vi "Angle PID.vi"(6 "reinitialize? (F)":bool, 7 "output range":cluster{"output high":dbl, "output low":dbl}={"output high"=100.0, "output low"=-100.0} {"output low" format="%.2f"; "output high" format="%.2f"}, 8 "dt (s)":dbl=-1.0 format="%.3f", 9 "PID gains":T1={"proportional gain (Kc)"=1.0, "integral time (Ti, min)"=0.01, "derivative time (Td, min)"=0.0} {"derivative time (Td, min)" format="%.3f"; "integral time (Ti, min)" format="%.3f"; "proportional gain (Kc)" format="%.3f"}, 10 "process variable":dbl format="%.2f", 11 "setpoint":dbl format="%.2f") -> (0 "dt out (s)":dbl format="%.3f", 3 "output":dbl format="%.2f")   [LabVIEW 2017]
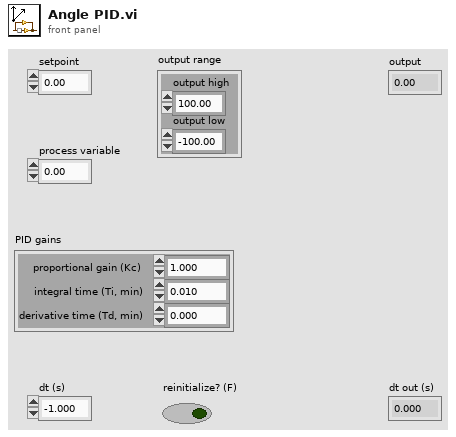
[diagram p1: front panel]
types:
  T1 = cluster{"proportional gain (Kc)":dbl, "integral time (Ti, min)":dbl, "derivative time (Td, min)":dbl}
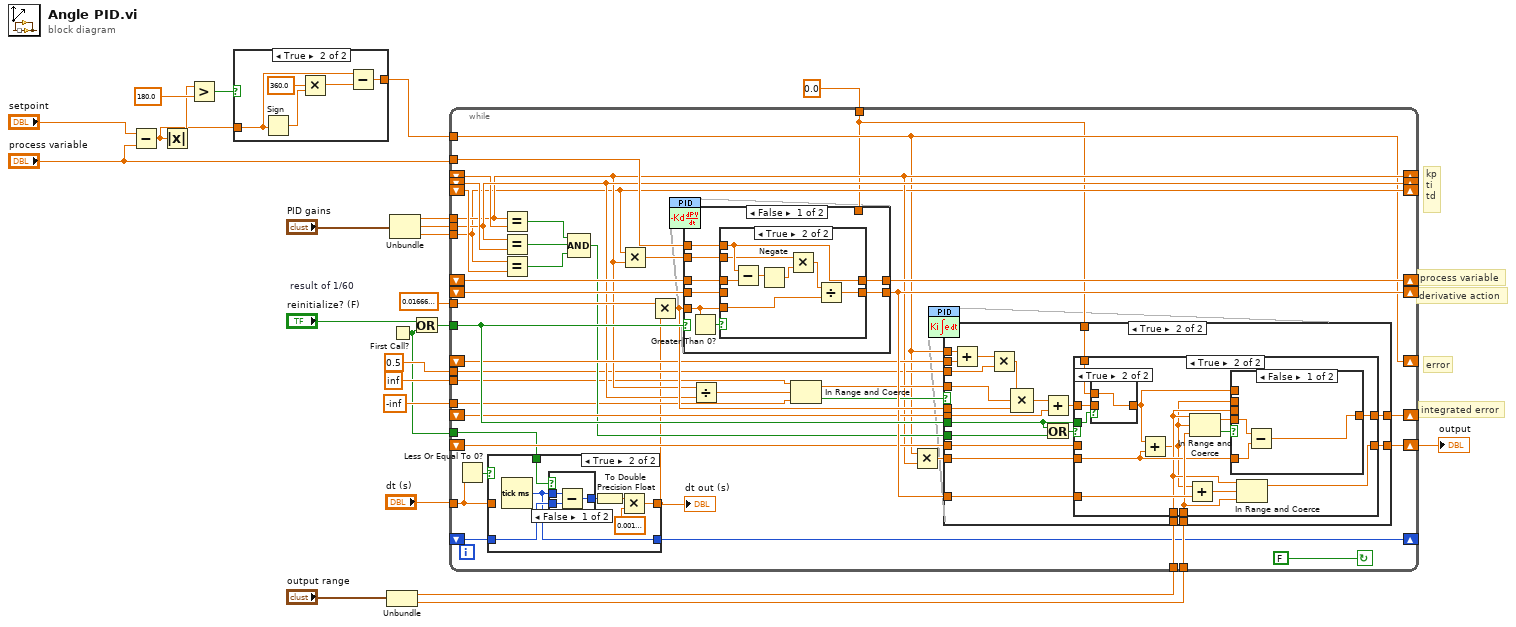
[diagram p0: block diagram]
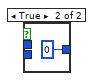
[diagram p4: hidden frame]
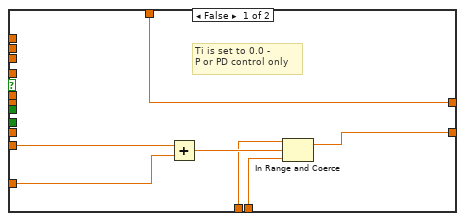
[diagram p5: hidden frame]
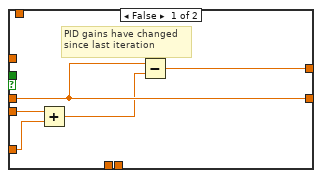
[diagram p6: hidden frame]
diagram:
  w18 = 0.016666666666666666  # result of 1/60
  # "derivative action"
  # "process variable"
  # "kp\nti\ntd"
  # "error"
  # "integrated error"
  n1 = Subtract(x="setpoint", y="process variable") -> (x-y=w2:dbl)
  n2 = Absolute Value(x=w2) -> (abs(x)=w4:dbl)
  n3 = Greater?(x=w4, y=180.0) -> (0:w3:bool)
  n4 = case shown="True" w3 {
    tunnel: w2 -> [w25 w28]
    tunnel: [w25 w26] -> w1
    frame False {
    }
    frame True {
      n5 = Sign(1:w28) -> (0:w29:dbl)
      n6 = Multiply(x=360.0, y=w29) -> (x*y=w30:dbl)
      n7 = Subtract(x=w28, y=w30) -> (x-y=w26:dbl)
    }
  }
  n8 = Unbundle("output range") -> ("output high"=w20:dbl, "output low"=w19:dbl)
  n9 = First Call?() -> (First Call?: T/F=w6:bool)
  n10 = Unbundle("PID gains") -> ("proportional gain (Kc)"=w23:dbl, "integral time (Ti, min)"=w22:dbl, "derivative time (Td, min)"=w21:dbl)
  n11 = Or(x="reinitialize? (F)", y=w6) -> (x .or. y?=w24:bool)
  n12 = while {
    tunnel: w24 -> [w72]
    shift-left: _ -> [w34]
    shift-right: [w35] -> _
    shift-right: [w44] -> _
    shift-left: _ -> [w45]
    shift-right: [w46] -> _
    shift-left: _ -> [w69]
    shift-right: [w39] -> _
    shift-left: _ -> [w70]
    tunnel: w23 -> [w44]
    tunnel: w22 -> [w46]
    tunnel: w21 -> [w39]
    tunnel: "dt (s)" -> [w33]
    tunnel: w20 -> [w65]
    tunnel: w19 -> [w64]
    tunnel: "process variable" -> [w63]
    shift-right: [w62] -> _
    shift-left: _ -> [w61]
    shift-right: [w60] -> _
    shift-left: _ -> [w52]
    shift-right: [w59] -> w11
    shift-left: _ -> [w58]
    shift-right: [w38] -> _
    shift-left: _ -> [w57]
    shift-right: [w56] -> _
    shift-left: _ -> [w55]
    tunnel: w18 -> [w49]
    tunnel: 0.5 ("y") -> [w43]
    tunnel: inf ("upper limit") -> [w41]
    tunnel: -inf ("lower limit") -> [w42]
    tunnel: w1 -> [w38]
    tunnel: 0.0 -> [w37]
    tunnel: w6 -> [w31]
    stop <- FALSE continue-if-true
    n13 = Less Or Equal To 0?(x=w33) -> (x <= 0?=w32:bool)
    n14 = case shown="True" w32 {
      tunnel: [w74 w78] -> w36
      tunnel: w34 -> [w73 w77]
      tunnel: [w73 w76] -> w35
      tunnel: w33 -> [w74 _]
      tunnel: w31 -> [_ w75]
      frame False {
      }
      frame True {
        n15 = Tick Count (ms)() -> (millisecond timer value=w76:u32)
        n16 = case shown="False" w75 {
          tunnel: [w84 u32 0] -> w80
          tunnel: w77 -> [w83 _]
          tunnel: w76 -> [w82 _]
          frame False {
            n17 = Subtract(x=w82, y=w83) -> (x-y=w84:u32)
          }
          frame True {
          }
        }
        n18 = To Double Precision Float(number=w80) -> (double precision float=w79:dbl)
        n19 = Multiply(x=w79, y=0.0010000000474974513) -> (x*y=w78:dbl)
      }
    }
    "dt out (s)" <- w36
    n20 = Equal?(x=w44, y=w45) -> (x = y?=w67:bool)
    n21 = Equal?(x=w46, y=w69) -> (x = y?=w66:bool)
    n22 = Equal?(x=w39, y=w70) -> (x = y?=w68:bool)
    n23 = Compound Arithmetic op=AND(w67, w66, w68) -> (w47:bool)
    n24 = Multiply(x=w39, y=w44) -> (x*y=w51:dbl)
    n25 = Multiply(x=w49, y=w36) -> (x*y=w71:dbl)
    n26 = case shown="False" w72 {
      tunnel: w61 -> [w146 _]
      tunnel: w51 -> [w143 _]
      tunnel: w63 -> [w145 w158]
      tunnel: [w142 w158] -> w62
      tunnel: [w144 w157] -> w60
      tunnel: w52 -> [w140 _]
      tunnel: w71 -> [w139 _]
      tunnel: w37 -> [_ w157]
      frame False {
        n27 = Greater Than 0?(x=w139) -> (x > 0?=w141:bool)
        n28 = case shown="True" w141 {
          tunnel: w146 -> [w148 w154]
          tunnel: w139 -> [_ w153]
          tunnel: w145 -> [_ w151]
          tunnel: [w147 w152] -> w144
          tunnel: w143 -> [_ w149]
          tunnel: [w148 w151] -> w142
          tunnel: w140 -> [w147 _]
          frame False {
            # "dt = 0 min"
          }
          frame True {
            n29 = Subtract(x=w151, y=w154) -> (x-y=w156:dbl)
            n30 = Negate(x=w156) -> (-x=w150:dbl)
            n31 = Multiply(x=w149, y=w150) -> (x*y=w155:dbl)
            n32 = Divide(x=w155, y=w153) -> (x/y=w152:dbl)
          }
        }
      }
      frame True {
      }
    }
    n33 = Divide(x=w44, y=w46) -> (x/y=w50:dbl)
    n34 = In Range and Coerce(upper limit=w41, x=w50, lower limit=w42) -> (coerced(x)=w54:dbl, In Range?=w53:bool)
    n35 = Multiply(x=w38, y=w44) -> (x*y=w48:dbl)
    n36 = case shown="True" w53 {
      tunnel: w38 -> [_ w112]
      tunnel: w57 -> [_ w113]
      tunnel: w55 -> [_ w108]
      tunnel: [w86 w103] -> w56
      tunnel: w54 -> [_ w101]
      tunnel: w48 -> [w91 w106]
      tunnel: [w92 w102] -> w59
      tunnel: w58 -> [_ w104]
      tunnel: w60 -> [w90 w100]
      tunnel: w72 -> [_ w99]
      tunnel: w47 -> [_ w98]
      tunnel: w71 -> [_ w97]
      tunnel: w65 -> [w88 w95]
      tunnel: w64 -> [w87 w96]
      tunnel: w43 -> [_ w94]
      tunnel: w37 -> [w86 w93]
      frame False {
        # "Ti is set to 0.0 -\nP or PD control only"
        n37 = Add(x=w91, y=w90) -> (x+y=w89:dbl)
        n38 = In Range and Coerce(upper limit=w88, x=w89, lower limit=w87) -> (coerced(x)=w92:dbl)  [unwired: 1 out]
      }
      frame True {
        n39 = Add(x=w112, y=w113) -> (x+y=w111:dbl)
        n40 = Multiply(x=w111, y=w94) -> (x*y=w110:dbl)
        n41 = Compound Arithmetic op=MULTIPLY(w110, w101, w97) -> (w109:dbl)
        n42 = Add(x=w109, y=w108) -> (x+y=w107:dbl)
        n43 = Or(x=w99, y=w98) -> (x .or. y?=w105:bool)
        n44 = case shown="True" w105 {
          tunnel: w107 -> [_ w126]
          tunnel: w106 -> [w116 w121]
          tunnel: w104 -> [w118 _]
          tunnel: w99 -> [_ w128]
          tunnel: [w117 w123] -> w103
          tunnel: [w118 w131] -> w102
          tunnel: w100 -> [w115 w130]
          tunnel: w96 -> [_ w129]
          tunnel: w95 -> [_ w120]
          tunnel: w93 -> [_ w127]
          frame False {
            # "PID gains have changed\nsince last iteration"
            n45 = Add(x=w116, y=w115) -> (x+y=w114:dbl)
            n46 = Subtract(x=w118, y=w114) -> (x-y=w117:dbl)
          }
          frame True {
            n47 = case shown="True" w128 {
              tunnel: w127 -> [_ w138]
              tunnel: [w137 w138] -> w125
              tunnel: w126 -> [w137 _]
              frame False {
              }
              frame True {
              }
            }
            n48 = Add(x=w125, y=w121) -> (x+y=w119:dbl)
            n49 = Add(x=w119, y=w130) -> (x+y=w132:dbl)
            n50 = In Range and Coerce(upper limit=w120, x=w119, lower limit=w129) -> (coerced(x)=w122:dbl, In Range?=w124:bool)
            n51 = case shown="False" w124 {
              tunnel: w125 -> [_ w136]
              tunnel: [w133 w136] -> w123
              tunnel: w122 -> [w135 _]
              tunnel: w121 -> [w134 _]
              tunnel: w120 -> [_ _]
              tunnel: w119 -> [_ _]
              frame False {
                n52 = Subtract(x=w135, y=w134) -> (x-y=w133:dbl)
              }
              frame True {
              }
            }
            n53 = In Range and Coerce(upper limit=w120, x=w132, lower limit=w129) -> (coerced(x)=w131:dbl)  [unwired: 1 out]
          }
        }
      }
    }
  }
  "output" <- w11
